vi "qSVO.vi"(0 "System no.":i32=1 min=1 max=4 step=1, 2 "Axes to query":string[](array[string]), 3 "All axes?":bool, 4 "Axis identifier?":bool=TRUE, 5 "error in":errorcluster) -> (14 "Servo status?":bool[](array[boolean]), 19 "error out":errorcluster)   [LabVIEW 2026]
doc: "GCS 3.0\n=====\n\nSVO? (Get Servo Mode) \n\nDescription\nQueries whether the current mode of operation of the axis is 0x2.\nFor further details on the modes of operation, see \"Drive State Machine\" (p. 101). \n\nFormat\nSVO?[ <AxisID>]\n\nArguments\nSVO? without arguments queries all axes of the controller.\n<AxisID>\nAn axis of the controller\nThe available axes can be queried with USG? SYS.\nPossible values: Alias of the axis (p. 94) \n\nResponse\n{<AxisID>\"=\"<Value>LF}\n<Value>\nValue that indicates the mode of operation of the axis\nPossible values:\n0 -> A mode of operation ? 0x2 Closed-Loop Position\n1 -> 0x2 Closed-Loop Position\n\nExample\n>>svo?\n<<AXIS_1=1\n<<AXIS_2=0\n>>sam?\n<<AXIS_1=0x2\n<<AXIS_2=0x0\n\nNotes\nThe current mode of operation of the axis is also displayed as follows:\n- In the status register of the axis (p. 97), which can be queried with the STV? command\n(p. 66) \n- Query with the SAM? command (p. 54) \nThe SVO command (p. 67) can be used to set the modes of operation 0x1 and 0x2.\nThe SAM command (p. 52) can be used to set all modes of operation supported for the axis.\n\nUser command level\nUSR\n\n\nGCS 2.0\n=====\n\nReturns servo status of queried axes.\n\nC-843, C-843.PM, C-844: If All axes? = TRUE, then Axis identifier? must be TRUE\n\nC-865, C-866: If All axes? = TRUE, then Axis identifier? must be TRUE\n\nE-516, E-710: If All axes? = TRUE, then Axis identifier? must be TRUE \n\nE-816: All axes? = FALSE, only one axis per command allowed.\n\nC-887, F-206, M-8X0: For GCS syntax version = GCS 1.0 (check with CSV?.vi. If CSV?.vi is not supported, syntax version is GCS 1.0), only first field of servo status array is valid. All axes? = TRUE, Axis identifier? = FALSE. \n\nAll other systems: If All axes? = TRUE, then Axis identifier? can be FALSE"
panel:
  # "SVO? (Get Servo Mode) \n\nQueries whether the current mode of operation of the axis is 0x2.\nFor further details on the modes of operation, see \"Drive State Machine\"."
  # "If all axes: use"
  # "Query"
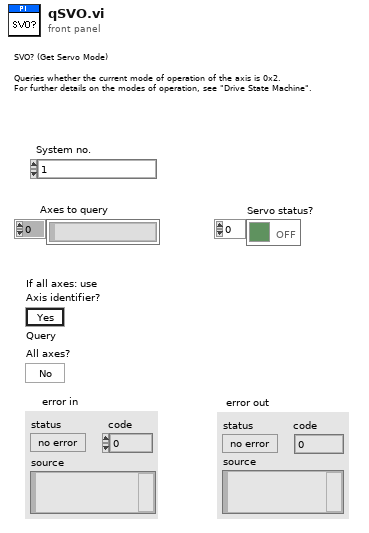
[diagram p1: front panel]
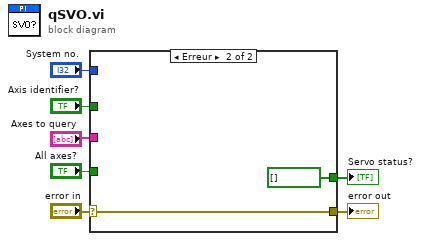
[diagram p0: block diagram]
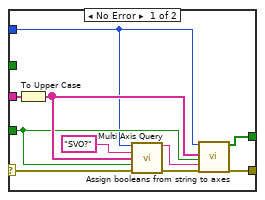
[diagram p2: hidden frame]
diagram:
  n1 = case shown="Erreur" "error in" {
    selector: "error in" -> [w16 w19]
    tunnel: [w11 bool[] [] ("Booleans")] -> w1
    tunnel: "Axes to query" -> [w17 _]
    tunnel: [w13 w19] -> w2
    tunnel: "System no." -> [w8 _]
    tunnel: "All axes?" -> [w9 _]
    tunnel: "Axis identifier?" -> [_ _]
    frame No Error {
      n2 = To Upper Case(1:w17) -> (0:w12:string[])
      n3 = call "Multi Axis Query.vi"("System no."=w8, "Command"="SVO?", "Axis"=w12, "All axes?"=w9, "error in (no error)"=w16) -> ("Answer"=w10:string, "error out"=w14:errorcluster)  [unwired: 9 in]
      n4 = call "Assign booleans from string to axes.vi"("System no."=w8, "Queried axes"=w12, "All axes queried?"=w9, "Input String"=w10, "error in"=w14) -> ("Booleans"=w11:bool[], "error out"=w13:errorcluster)  [unwired: 13 in]
    }
    frame Error {
      (unwired) string[] [] ("Axes to query out")
    }
  }
  "error out" <- w2
  "Servo status?" <- w1
